vi "Parse Event String.vi"(8 "error in (no error)":errorcluster, 10 "Message":string) -> (0 "error out":errorcluster, 1 "Valid?":bool, 2 "Event":T1)   [LabVIEW 2019, in "Muon Detector.lvclass"]
uses:
  Muon Detector.lvclass
  Event.ctl
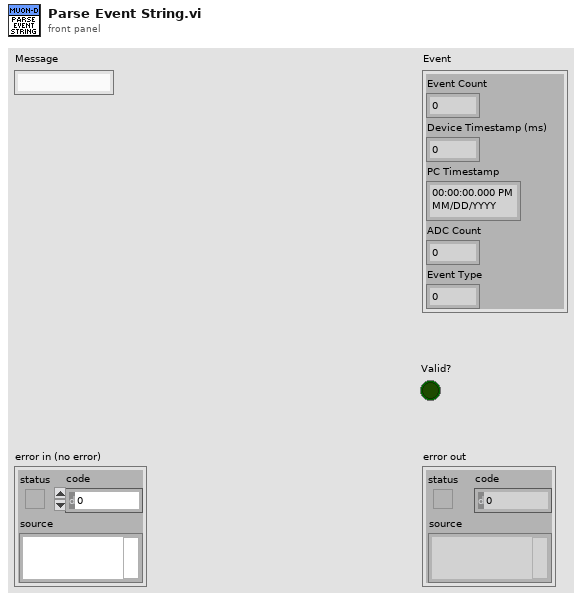
[diagram p1: front panel]
types:
  T1 = typedef "Muon Detector.lvclass/Event.ctl" = cluster{"Event Count":i32, "Device Timestamp (ms)":i32, "PC Timestamp":timestamp, "ADC Count":i32, "Event Type":u8}
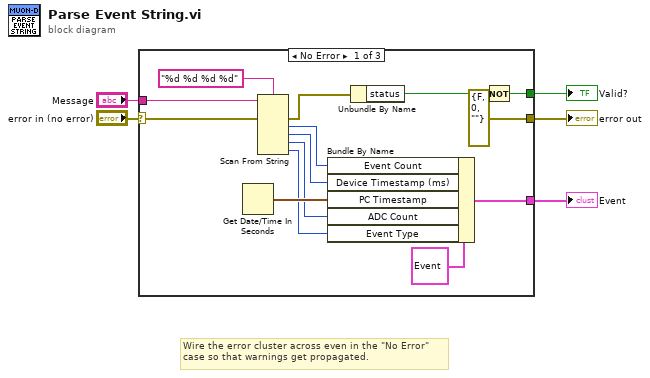
[diagram p0: block diagram]
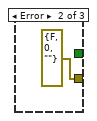
[diagram p2: hidden frame]
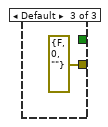
[diagram p3: hidden frame]
diagram:
  # "Wire the error cluster across even in the \"No Error\"\ncase so that warnings get propagated."
  n1 = case shown="No Error" "error in (no error)" {
    selector: "error in (no error)" -> [w8 _ _]
    tunnel: [errorcluster {"status"=FALSE, "code"=0, "source"=""} ("error IO") errorcluster {"status"=FALSE, "code"=0, "source"=""} ("error IO") errorcluster {"status"=FALSE, "code"=0, "source"=""} ("error IO")] -> w4
    tunnel: "Message" -> [w16 _ _]
    tunnel: [w10 _ _] -> w2
    tunnel: [w9 _ _] -> w1
    frame No Error {
      n2 = Get Date/Time In Seconds() -> (seconds since 1Jan1904=w14:timestamp)
      n3 = Scan From String(format string="%d %d %d %d", input string=w16, error in=w8) -> (error out=w7:errorcluster, output 1=w18:i32, output 2=w17:i32, output 3=w13:i32, output 4=w12:i32)  [unwired: 5 in, 2 out]
      n4 = Bundle By Name(cluster=T1 {"Event Count"=0, "Device Timestamp (ms)"=0, "PC Timestamp"=timestamp(0 s since 1904-01-01), "ADC Count"=0, "Event Type"=0} ("Event"), "Event Count"=w18, "Device Timestamp (ms)"=w17, "PC Timestamp"=w14, "ADC Count"=w13, "Event Type"=w12) -> (w9:T1)
      n5 = Unbundle By Name(w7) -> ("status"=w11:bool)
      n6 = Not(x=w11) -> (.not. x?=w10:bool)
    }
    frame Error {
    }
    frame Default {
    }
  }
  "error out" <- w4
  "Event" <- w1
  "Valid?" <- w2
